vi "HMI-BPCS-RX.vi"(0 "Digital in":refnum<vi>, 1 "DigNum Refnum 9":refnum<vi>, 2 "DigNum Refnum":refnum<vi>, 3 "reference 10":refnum<vi>, 4 "reference 2":refnum<vi>, 5 "DigNum Refnum 8":refnum<vi>, 6 "Bool Refnum 2":refnum<vi>, 8 "reference":refnum<vi>, 9 "reference 9":refnum<vi>, 10 "Bool Refnum":refnum<vi>, 11 "reference 3":refnum<vi>, 12 "DigNum Refnum 10":refnum<vi>, 13 "DigNum Refnum 7":refnum<vi>, 14 "reference 12":refnum<vi>, 15 "DigNum Refnum 2":refnum<vi>, 16 "DigNum Refnum 11":refnum<vi>, 17 "reference 8":refnum<vi>, 18 "reference 13":refnum<vi>, 19 "reference 4":refnum<vi>, 21 "DigNum Refnum 6":refnum<vi>, 22 "reference 7":refnum<vi>, 23 "DigNum Refnum 5":refnum<vi>, 24 "reference 6":refnum<vi>, 25 "DigNum Refnum 4":refnum<vi>, 26 "reference 5":refnum<vi>, 27 "DigNum Refnum 3":refnum<vi>) -> ()   [LabVIEW 2018]
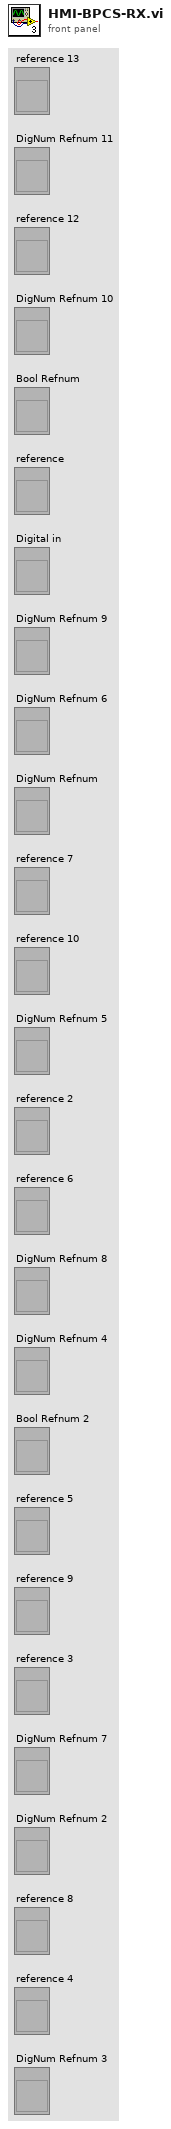
[diagram p1: front panel]
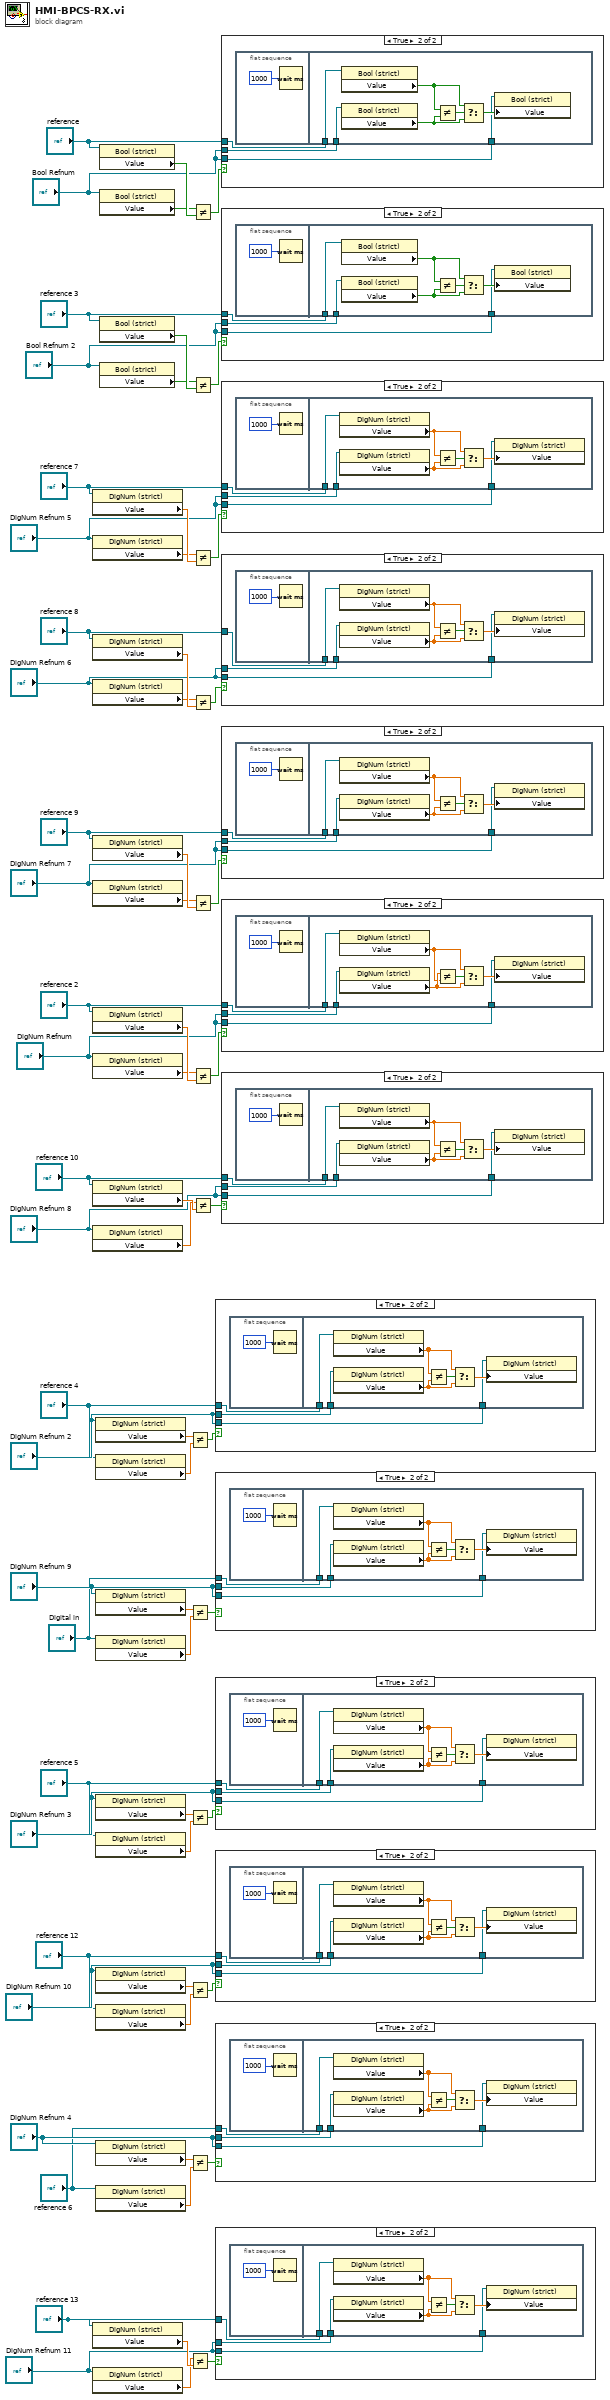
[diagram p0: block diagram]
diagram:
  n1 = property class="DigNum (strict)"(reference="reference 7") -> ("Value"=w47:dbl)  [unwired: 1 in, 2 out]
  n2 = property on="Property Node" class="DigNum (strict)"(reference="DigNum Refnum 5") -> ("Value"=w46:dbl)  [unwired: 1 in, 2 out]
  n3 = property class="DigNum (strict)"(reference="reference 8") -> ("Value"=w50:dbl)  [unwired: 1 in, 2 out]
  n4 = property on="Property Node" class="DigNum (strict)"(reference="DigNum Refnum 6") -> ("Value"=w49:dbl)  [unwired: 1 in, 2 out]
  n5 = property class="DigNum (strict)"(reference="reference 9") -> ("Value"=w53:dbl)  [unwired: 1 in, 2 out]
  n6 = property on="Property Node" class="DigNum (strict)"(reference="DigNum Refnum 7") -> ("Value"=w52:dbl)  [unwired: 1 in, 2 out]
  n7 = property class="DigNum (strict)"(reference="reference 2") -> ("Value"=w32:dbl)  [unwired: 1 in, 2 out]
  n8 = property on="Property Node" class="DigNum (strict)"(reference="DigNum Refnum") -> ("Value"=w31:dbl)  [unwired: 1 in, 2 out]
  n9 = property class="DigNum (strict)"(reference="reference 10") -> ("Value"=w55:dbl)  [unwired: 1 in, 2 out]
  n10 = property on="Property Node" class="DigNum (strict)"(reference="DigNum Refnum 8") -> ("Value"=w54:dbl)  [unwired: 1 in, 2 out]
  n11 = property class="DigNum (strict)"(reference="reference 13") -> ("Value"=w65:dbl)  [unwired: 1 in, 2 out]
  n12 = property on="Property Node" class="DigNum (strict)"(reference="DigNum Refnum 11") -> ("Value"=w64:dbl)  [unwired: 1 in, 2 out]
  n13 = property on="Property Node" class="DigNum (strict)"(reference="DigNum Refnum 2") -> ("Value"=w37:dbl)  [unwired: 1 in, 2 out]
  n14 = property class="DigNum (strict)"(reference="reference 4") -> ("Value"=w38:dbl)  [unwired: 1 in, 2 out]
  n15 = property on="Property Node" class="DigNum (strict)"(reference="DigNum Refnum 9") -> ("Value"=w58:dbl)  [unwired: 1 in, 2 out]
  n16 = property class="DigNum (strict)"(reference="Digital in") -> ("Value"=w59:dbl)  [unwired: 1 in, 2 out]
  n17 = property on="Property Node" class="DigNum (strict)"(reference="DigNum Refnum 3") -> ("Value"=w40:dbl)  [unwired: 1 in, 2 out]
  n18 = property class="DigNum (strict)"(reference="reference 5") -> ("Value"=w41:dbl)  [unwired: 1 in, 2 out]
  n19 = property on="Property Node" class="DigNum (strict)"(reference="DigNum Refnum 10") -> ("Value"=w62:dbl)  [unwired: 1 in, 2 out]
  n20 = property class="DigNum (strict)"(reference="reference 12") -> ("Value"=w63:dbl)  [unwired: 1 in, 2 out]
  n21 = property on="Property Node" class="DigNum (strict)"(reference="DigNum Refnum 4") -> ("Value"=w43:dbl)  [unwired: 1 in, 2 out]
  n22 = property class="DigNum (strict)"(reference="reference 6") -> ("Value"=w44:dbl)  [unwired: 1 in, 2 out]
  n23 = property class="Bool (strict)"(reference="reference") -> ("Value"=w29:bool)  [unwired: 1 in, 2 out]
  n24 = property on="Property Node" class="Bool (strict)"(reference="Bool Refnum") -> ("Value"=w28:bool)  [unwired: 1 in, 2 out]
  n25 = property class="Bool (strict)"(reference="reference 3") -> ("Value"=w35:bool)  [unwired: 1 in, 2 out]
  n26 = property on="Property Node" class="Bool (strict)"(reference="Bool Refnum 2") -> ("Value"=w34:bool)  [unwired: 1 in, 2 out]
  n27 = Not Equal?(x=w37, y=w38) -> (x != y?=w36:bool)
  n28 = Not Equal?(x=w58, y=w59) -> (x != y?=w57:bool)
  n29 = Not Equal?(x=w40, y=w41) -> (x != y?=w39:bool)
  n30 = Not Equal?(x=w62, y=w63) -> (x != y?=w60:bool)
  n31 = Not Equal?(x=w43, y=w44) -> (x != y?=w42:bool)
  n32 = Not Equal?(x=w64, y=w65) -> (x != y?=w61:bool)
  n33 = Not Equal?(x=w28, y=w29) -> (x != y?=w27:bool)
  n34 = Not Equal?(x=w34, y=w35) -> (x != y?=w33:bool)
  n35 = Not Equal?(x=w46, y=w47) -> (x != y?=w45:bool)
  n36 = Not Equal?(x=w49, y=w50) -> (x != y?=w48:bool)
  n37 = Not Equal?(x=w52, y=w53) -> (x != y?=w51:bool)
  n38 = Not Equal?(x=w31, y=w32) -> (x != y?=w30:bool)
  n39 = Not Equal?(x=w54, y=w55) -> (x != y?=w56:bool)
  n40 = case shown="True" w36 {
    tunnel: "DigNum Refnum 2" -> [_ w68]
    tunnel: "DigNum Refnum 2" -> [_ w67]
    tunnel: "reference 4" -> [_ w66]
    frame False {
    }
    frame True {
      n41 = flat-sequence {
        tunnel: w68 -> [w72]
        tunnel: w67 -> [w71]
        tunnel: w66 -> [w70]
        frame #0 {
          n42 = Wait (ms)(milliseconds to wait=u32 1000) -> ()  [unwired: 1 out]
        }
        frame #1 {
          n43 = property class="DigNum (strict)"(reference=w70) -> ("Value"=w74:dbl)  [unwired: 1 in, 2 out]
          n44 = property on="Property Node" class="DigNum (strict)"(reference=w72) -> ("Value"=w73:dbl)  [unwired: 1 in, 2 out]
          n45 = Not Equal?(x=w74, y=w73) -> (x != y?=w76:bool)
          n46 = Select(t=w74, s=w76, f=w73) -> (s? t:f=w75:dbl)
          n47 = property on="Property Node" class="DigNum (strict)"(reference=w71, "Value"=w75) -> ()  [unwired: 1 in, 2 out]
        }
      }
    }
  }
  n48 = case shown="True" w57 {
    tunnel: "DigNum Refnum 9" -> [_ w79]
    tunnel: "DigNum Refnum 9" -> [_ w78]
    tunnel: "Digital in" -> [_ w77]
    frame False {
    }
    frame True {
      n49 = flat-sequence {
        tunnel: w79 -> [w83]
        tunnel: w78 -> [w82]
        tunnel: w77 -> [w81]
        frame #0 {
          n50 = Wait (ms)(milliseconds to wait=u32 1000) -> ()  [unwired: 1 out]
        }
        frame #1 {
          n51 = property class="DigNum (strict)"(reference=w81) -> ("Value"=w86:dbl)  [unwired: 1 in, 2 out]
          n52 = property on="Property Node" class="DigNum (strict)"(reference=w82) -> ("Value"=w85:dbl)  [unwired: 1 in, 2 out]
          n53 = Not Equal?(x=w86, y=w85) -> (x != y?=w87:bool)
          n54 = Select(t=w86, s=w87, f=w85) -> (s? t:f=w84:dbl)
          n55 = property on="Property Node" class="DigNum (strict)"(reference=w83, "Value"=w84) -> ()  [unwired: 1 in, 2 out]
        }
      }
    }
  }
  n56 = case shown="True" w39 {
    tunnel: "DigNum Refnum 3" -> [_ w90]
    tunnel: "DigNum Refnum 3" -> [_ w89]
    tunnel: "reference 5" -> [_ w88]
    frame False {
    }
    frame True {
      n57 = flat-sequence {
        tunnel: w90 -> [w94]
        tunnel: w89 -> [w93]
        tunnel: w88 -> [w92]
        frame #0 {
          n58 = Wait (ms)(milliseconds to wait=u32 1000) -> ()  [unwired: 1 out]
        }
        frame #1 {
          n59 = property class="DigNum (strict)"(reference=w92) -> ("Value"=w96:dbl)  [unwired: 1 in, 2 out]
          n60 = property on="Property Node" class="DigNum (strict)"(reference=w94) -> ("Value"=w95:dbl)  [unwired: 1 in, 2 out]
          n61 = Not Equal?(x=w96, y=w95) -> (x != y?=w98:bool)
          n62 = Select(t=w96, s=w98, f=w95) -> (s? t:f=w97:dbl)
          n63 = property on="Property Node" class="DigNum (strict)"(reference=w93, "Value"=w97) -> ()  [unwired: 1 in, 2 out]
        }
      }
    }
  }
  n64 = case shown="True" w60 {
    tunnel: "DigNum Refnum 10" -> [_ w101]
    tunnel: "DigNum Refnum 10" -> [_ w100]
    tunnel: "reference 12" -> [_ w99]
    frame False {
    }
    frame True {
      n65 = flat-sequence {
        tunnel: w101 -> [w105]
        tunnel: w100 -> [w104]
        tunnel: w99 -> [w103]
        frame #0 {
          n66 = Wait (ms)(milliseconds to wait=u32 1000) -> ()  [unwired: 1 out]
        }
        frame #1 {
          n67 = property class="DigNum (strict)"(reference=w103) -> ("Value"=w107:dbl)  [unwired: 1 in, 2 out]
          n68 = property on="Property Node" class="DigNum (strict)"(reference=w105) -> ("Value"=w106:dbl)  [unwired: 1 in, 2 out]
          n69 = Not Equal?(x=w107, y=w106) -> (x != y?=w109:bool)
          n70 = Select(t=w107, s=w109, f=w106) -> (s? t:f=w108:dbl)
          n71 = property on="Property Node" class="DigNum (strict)"(reference=w104, "Value"=w108) -> ()  [unwired: 1 in, 2 out]
        }
      }
    }
  }
  n72 = case shown="True" w42 {
    tunnel: "DigNum Refnum 4" -> [_ w112]
    tunnel: "DigNum Refnum 4" -> [_ w111]
    tunnel: "reference 6" -> [_ w110]
    frame False {
    }
    frame True {
      n73 = flat-sequence {
        tunnel: w112 -> [w116]
        tunnel: w111 -> [w115]
        tunnel: w110 -> [w114]
        frame #0 {
          n74 = Wait (ms)(milliseconds to wait=u32 1000) -> ()  [unwired: 1 out]
        }
        frame #1 {
          n75 = property class="DigNum (strict)"(reference=w114) -> ("Value"=w118:dbl)  [unwired: 1 in, 2 out]
          n76 = property on="Property Node" class="DigNum (strict)"(reference=w115) -> ("Value"=w117:dbl)  [unwired: 1 in, 2 out]
          n77 = Not Equal?(x=w118, y=w117) -> (x != y?=w120:bool)
          n78 = Select(t=w118, s=w120, f=w117) -> (s? t:f=w119:dbl)
          n79 = property on="Property Node" class="DigNum (strict)"(reference=w116, "Value"=w119) -> ()  [unwired: 1 in, 2 out]
        }
      }
    }
  }
  n80 = case shown="True" w61 {
    tunnel: "DigNum Refnum 11" -> [_ w123]
    tunnel: "DigNum Refnum 11" -> [_ w122]
    tunnel: "reference 13" -> [_ w121]
    frame False {
    }
    frame True {
      n81 = flat-sequence {
        tunnel: w123 -> [w127]
        tunnel: w122 -> [w126]
        tunnel: w121 -> [w125]
        frame #0 {
          n82 = Wait (ms)(milliseconds to wait=u32 1000) -> ()  [unwired: 1 out]
        }
        frame #1 {
          n83 = property class="DigNum (strict)"(reference=w125) -> ("Value"=w129:dbl)  [unwired: 1 in, 2 out]
          n84 = property on="Property Node" class="DigNum (strict)"(reference=w127) -> ("Value"=w128:dbl)  [unwired: 1 in, 2 out]
          n85 = Not Equal?(x=w129, y=w128) -> (x != y?=w131:bool)
          n86 = Select(t=w129, s=w131, f=w128) -> (s? t:f=w130:dbl)
          n87 = property on="Property Node" class="DigNum (strict)"(reference=w126, "Value"=w130) -> ()  [unwired: 1 in, 2 out]
        }
      }
    }
  }
  n88 = case shown="True" w27 {
    tunnel: "Bool Refnum" -> [_ w134]
    tunnel: "reference" -> [_ w133]
    tunnel: "Bool Refnum" -> [_ w132]
    frame False {
    }
    frame True {
      n89 = flat-sequence {
        tunnel: w134 -> [w138]
        tunnel: w133 -> [w137]
        tunnel: w132 -> [w136]
        frame #0 {
          n90 = Wait (ms)(milliseconds to wait=u32 1000) -> ()  [unwired: 1 out]
        }
        frame #1 {
          n91 = property class="Bool (strict)"(reference=w137) -> ("Value"=w140:bool)  [unwired: 1 in, 2 out]
          n92 = property on="Property Node" class="Bool (strict)"(reference=w138) -> ("Value"=w139:bool)  [unwired: 1 in, 2 out]
          n93 = Not Equal?(x=w140, y=w139) -> (x != y?=w142:bool)
          n94 = Select(t=w140, s=w142, f=w139) -> (s? t:f=w141:bool)
          n95 = property on="Property Node" class="Bool (strict)"(reference=w136, "Value"=w141) -> ()  [unwired: 1 in, 2 out]
        }
      }
    }
  }
  n96 = case shown="True" w33 {
    tunnel: "Bool Refnum 2" -> [_ w145]
    tunnel: "Bool Refnum 2" -> [_ w144]
    tunnel: "reference 3" -> [_ w143]
    frame False {
    }
    frame True {
      n97 = flat-sequence {
        tunnel: w145 -> [w149]
        tunnel: w144 -> [w148]
        tunnel: w143 -> [w147]
        frame #0 {
          n98 = Wait (ms)(milliseconds to wait=u32 1000) -> ()  [unwired: 1 out]
        }
        frame #1 {
          n99 = property class="Bool (strict)"(reference=w147) -> ("Value"=w151:bool)  [unwired: 1 in, 2 out]
          n100 = property on="Property Node" class="Bool (strict)"(reference=w149) -> ("Value"=w150:bool)  [unwired: 1 in, 2 out]
          n101 = Not Equal?(x=w151, y=w150) -> (x != y?=w153:bool)
          n102 = Select(t=w151, s=w153, f=w150) -> (s? t:f=w152:bool)
          n103 = property on="Property Node" class="Bool (strict)"(reference=w148, "Value"=w152) -> ()  [unwired: 1 in, 2 out]
        }
      }
    }
  }
  n104 = case shown="True" w45 {
    tunnel: "DigNum Refnum 5" -> [_ w156]
    tunnel: "DigNum Refnum 5" -> [_ w155]
    tunnel: "reference 7" -> [_ w154]
    frame False {
    }
    frame True {
      n105 = flat-sequence {
        tunnel: w156 -> [w160]
        tunnel: w155 -> [w159]
        tunnel: w154 -> [w158]
        frame #0 {
          n106 = Wait (ms)(milliseconds to wait=u32 1000) -> ()  [unwired: 1 out]
        }
        frame #1 {
          n107 = property class="DigNum (strict)"(reference=w158) -> ("Value"=w162:dbl)  [unwired: 1 in, 2 out]
          n108 = property on="Property Node" class="DigNum (strict)"(reference=w160) -> ("Value"=w161:dbl)  [unwired: 1 in, 2 out]
          n109 = Not Equal?(x=w162, y=w161) -> (x != y?=w164:bool)
          n110 = Select(t=w162, s=w164, f=w161) -> (s? t:f=w163:dbl)
          n111 = property on="Property Node" class="DigNum (strict)"(reference=w159, "Value"=w163) -> ()  [unwired: 1 in, 2 out]
        }
      }
    }
  }
  n112 = case shown="True" w48 {
    tunnel: "DigNum Refnum 6" -> [_ w167]
    tunnel: "DigNum Refnum 6" -> [_ w166]
    tunnel: "reference 8" -> [_ w165]
    frame False {
    }
    frame True {
      n113 = flat-sequence {
        tunnel: w167 -> [w171]
        tunnel: w166 -> [w170]
        tunnel: w165 -> [w169]
        frame #0 {
          n114 = Wait (ms)(milliseconds to wait=u32 1000) -> ()  [unwired: 1 out]
        }
        frame #1 {
          n115 = property class="DigNum (strict)"(reference=w169) -> ("Value"=w173:dbl)  [unwired: 1 in, 2 out]
          n116 = property on="Property Node" class="DigNum (strict)"(reference=w170) -> ("Value"=w172:dbl)  [unwired: 1 in, 2 out]
          n117 = Not Equal?(x=w173, y=w172) -> (x != y?=w175:bool)
          n118 = Select(t=w173, s=w175, f=w172) -> (s? t:f=w174:dbl)
          n119 = property on="Property Node" class="DigNum (strict)"(reference=w171, "Value"=w174) -> ()  [unwired: 1 in, 2 out]
        }
      }
    }
  }
  n120 = case shown="True" w51 {
    tunnel: "DigNum Refnum 7" -> [_ w178]
    tunnel: "DigNum Refnum 7" -> [_ w177]
    tunnel: "reference 9" -> [_ w176]
    frame False {
    }
    frame True {
      n121 = flat-sequence {
        tunnel: w178 -> [w182]
        tunnel: w177 -> [w181]
        tunnel: w176 -> [w180]
        frame #0 {
          n122 = Wait (ms)(milliseconds to wait=u32 1000) -> ()  [unwired: 1 out]
        }
        frame #1 {
          n123 = property class="DigNum (strict)"(reference=w180) -> ("Value"=w184:dbl)  [unwired: 1 in, 2 out]
          n124 = property on="Property Node" class="DigNum (strict)"(reference=w182) -> ("Value"=w183:dbl)  [unwired: 1 in, 2 out]
          n125 = Not Equal?(x=w184, y=w183) -> (x != y?=w186:bool)
          n126 = Select(t=w184, s=w186, f=w183) -> (s? t:f=w185:dbl)
          n127 = property on="Property Node" class="DigNum (strict)"(reference=w181, "Value"=w185) -> ()  [unwired: 1 in, 2 out]
        }
      }
    }
  }
  n128 = case shown="True" w30 {
    tunnel: "DigNum Refnum" -> [_ w189]
    tunnel: "reference 2" -> [_ w188]
    tunnel: "DigNum Refnum" -> [_ w187]
    frame False {
    }
    frame True {
      n129 = flat-sequence {
        tunnel: w189 -> [w193]
        tunnel: w188 -> [w192]
        tunnel: w187 -> [w191]
        frame #0 {
          n130 = Wait (ms)(milliseconds to wait=u32 1000) -> ()  [unwired: 1 out]
        }
        frame #1 {
          n131 = property class="DigNum (strict)"(reference=w192) -> ("Value"=w194:dbl)  [unwired: 1 in, 2 out]
          n132 = property on="Property Node" class="DigNum (strict)"(reference=w193) -> ("Value"=w196:dbl)  [unwired: 1 in, 2 out]
          n133 = Not Equal?(x=w196, y=w194) -> (x != y?=w197:bool)
          n134 = Select(t=w194, s=w197, f=w196) -> (s? t:f=w195:dbl)
          n135 = property on="Property Node" class="DigNum (strict)"(reference=w191, "Value"=w195) -> ()  [unwired: 1 in, 2 out]
        }
      }
    }
  }
  n136 = case shown="True" w56 {
    tunnel: "DigNum Refnum 8" -> [_ w200]
    tunnel: "DigNum Refnum 8" -> [_ w199]
    tunnel: "reference 10" -> [_ w198]
    frame False {
    }
    frame True {
      n137 = flat-sequence {
        tunnel: w200 -> [w204]
        tunnel: w199 -> [w203]
        tunnel: w198 -> [w202]
        frame #0 {
          n138 = Wait (ms)(milliseconds to wait=u32 1000) -> ()  [unwired: 1 out]
        }
        frame #1 {
          n139 = property class="DigNum (strict)"(reference=w202) -> ("Value"=w206:dbl)  [unwired: 1 in, 2 out]
          n140 = property on="Property Node" class="DigNum (strict)"(reference=w204) -> ("Value"=w205:dbl)  [unwired: 1 in, 2 out]
          n141 = Not Equal?(x=w206, y=w205) -> (x != y?=w208:bool)
          n142 = Select(t=w206, s=w208, f=w205) -> (s? t:f=w207:dbl)
          n143 = property on="Property Node" class="DigNum (strict)"(reference=w203, "Value"=w207) -> ()  [unwired: 1 in, 2 out]
        }
      }
    }
  }
